vi "usrp get rx stream.vi"(8 "error in (no error)":errorcluster, 9 "h 3":u64, 10 "stream_args":T2, 11 "h":u64) -> (0 "error out":errorcluster, 1 "h 4":u64, 2 "stream_args 2":T1, 3 "h 2":u64, 4 "function return":u32(ring))   [LabVIEW 2023, in "uhd.lvlib"]
doc: "UHD_API uhd_error uhd_usrp_get_rx_stream(\n uhd_usrp_handle h, uhd_stream_args_t* stream_args, uhd_rx_streamer_handle h_out);"
uses:
  <userlib>/uhd/uhd.lvlib
  <userlib>/uhd/uhd.dll
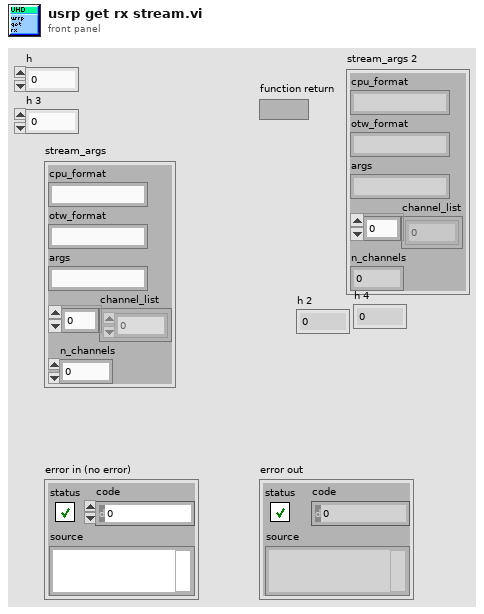
[diagram p1: front panel]
types:
  T1 = cluster{"cpu_format":string, "otw_format":string, "args":string, "channel_list":u64[], "n_channels":i32}
  T2 = cluster{"cpu_format":string, "otw_format":string, "args":string, "channel_list":u64[], "n_channels":u64}
  T3 = cluster{"cpu_format":u64, "otw_format":u64, "args":u64, "channel_list":u64, "n_channels":i32}
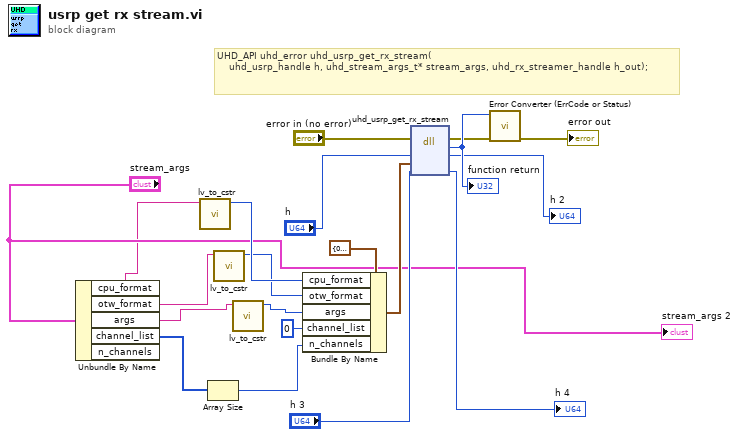
[diagram p0: block diagram]
diagram:
  # "UHD_API uhd_error uhd_usrp_get_rx_stream(\n    uhd_usrp_handle h, uhd_stream_args_t* stream_args, uhd_rx_streamer_handle h_out);"
  n1 = Unbundle By Name("stream_args") -> ("cpu_format"=w6:string, "otw_format"=w5:string, "args"=w3:string, "channel_list"=w7:u64[])  [unwired: 1 out]
  n2 = call <userlib>:"lv_to_cstr.vi"("cpu_format"=w6) -> ("CStrP"=w9:u64)  [unwired: 10 in]
  n3 = Array Size(array=w7) -> (size(s)=w15:i32)
  n4 = call <userlib>:"lv_to_cstr.vi"("cpu_format"=w5) -> ("CStrP"=w4:u64)  [unwired: 10 in]
  n5 = call <userlib>:"lv_to_cstr.vi"("cpu_format"=w3) -> ("CStrP"=w2:u64)  [unwired: 10 in]
  n6 = Bundle By Name(cluster=T3 {"cpu_format"=0, "otw_format"=0, "args"=0, "channel_list"=0, "n_channels"=0} ("stream_args"), "cpu_format"=w9, "otw_format"=w4, "args"=w2, "channel_list"=u64 0, "n_channels"=w15) -> (w19:T3)
  n7 = dll-call lib="C:/Program Files/National Instruments/LabVIEW 2023/user.lib/uhd/uhd.dll" fn="uhd_usrp_get_rx_stream"(error in="error in (no error)", "h"="h", "stream_args"=w19, "h_out"="h 3") -> (error out=w17:errorcluster, "return type"=w20:u32, "h"=→"h 2":u64, "h_out"=→"h 4":u64)  [unwired: 3 in, 1 out]
  "function return" <- w20
  n8 = call <userlib>:"Error Converter (ErrCode or Status).vi"("error in (no error)"=w17, "error code"=w20) -> ("error out"=→"error out":errorcluster)  [unwired: 9 in]
  "stream_args 2" <- "stream_args"
